vi "logEvent.vi"(8 "error in":errorcluster, 10 "event,data":string, 11 "fileRef":refnum<file>) -> (0 "error out":errorcluster)   [LabVIEW 2024]
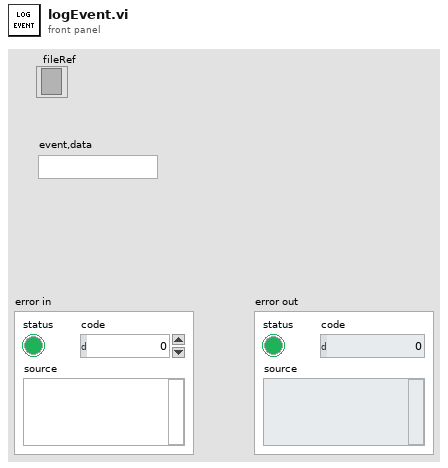
[diagram p1: front panel]
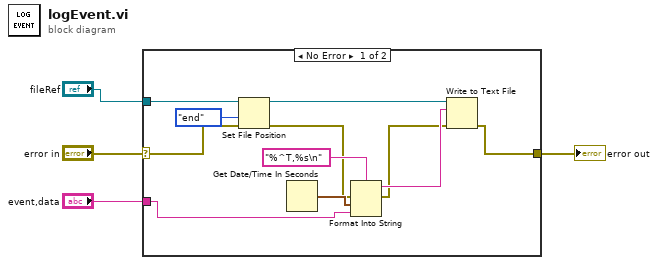
[diagram p0: block diagram]
diagram:
  n1 = case shown="No Error" "error in" {
    selector: "error in" -> [w15 w16]
    tunnel: [w12 w16] -> w3
    tunnel: "fileRef" -> [w14 _]
    tunnel: "event,data" -> [w6 _]
    frame No Error {
      n2 = Set File Position(refnum=w14, from (0:start)=enum16{"start", "end", "current"}."end", error in=w15) -> (refnum out=w13:refnum<file>, error out=w8:errorcluster)  [unwired: 1 in]
      n3 = Get Date/Time In Seconds() -> (seconds since 1Jan1904=w11:timestamp)
      n4 = Format Into String(format string="%^T,%s\n" ("text"), error in=w8, w11, w6) -> (resulting string=w9:string, error out=w7:errorcluster)  [unwired: 1 in]
      n5 = Write to Text File(file (use dialog)=w13, text=w9, error in=w7) -> (error out=w12:errorcluster)  [unwired: 1 in, 2 out]
    }
    frame Error {
    }
  }
  "error out" <- w3
